vi "GetRectUnion.vi"(8 "No Error":errorcluster, 10 "B":T1, 11 "A":T1) -> (0 "Error Out":errorcluster, 3 "Union":T1)   [LabVIEW 2024, in "SDL3.lvlib" / "Rect.lvlib"]
doc: "<B>Summary</B>\nCalculate the union of two rectangles."
uses:
  Rect.lvlib
  Rect--cluster.ctl
  Lib/SDL3.dll
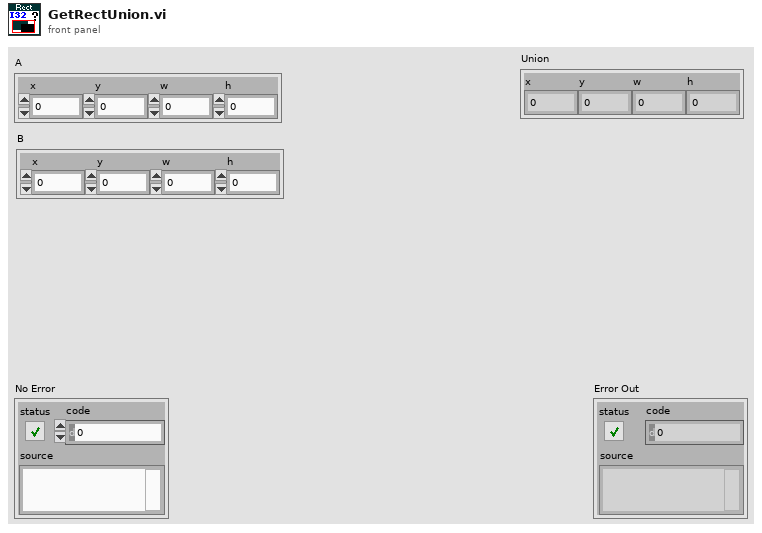
[diagram p1: front panel]
types:
  T1 = typedef "SDL3.lvlib/Rect.lvlib/Rect--cluster.ctl" = cluster{"x":i32, "y":i32, "w":i32, "h":i32}
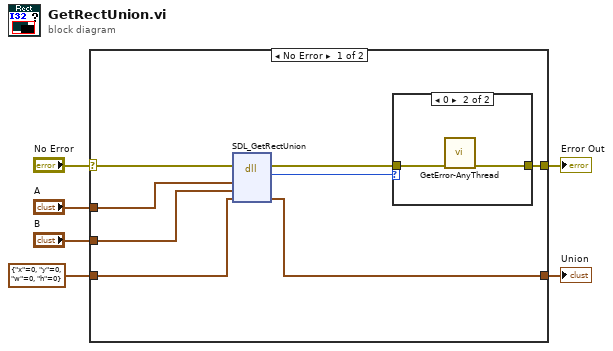
[diagram p0: block diagram]
diagram:
  n1 = case shown="No Error" "No Error" {
    selector: "No Error" -> [w14 w19]
    tunnel: "A" -> [w12 _]
    tunnel: "B" -> [w11 _]
    tunnel: [w10 w18] -> w3
    tunnel: [w9 w19] -> w2
    tunnel: T1 {"x"=0, "y"=0, "w"=0, "h"=0} ("B") -> [w7 w18]
    frame No Error {
      n2 = dll-call lib="C:/Users/Thomas/Documents/Projects/LV-SDL3/Sources/SDL3/Lib/SDL3.*" fn="SDL_GetRectUnion"(error in=w14, "A"=w12, "B"=w11, "result"=w7) -> (error out=w13:errorcluster, "return type"=w8:i32, "result"=w10:T1)  [unwired: 4 in, 1 out]
      n3 = case shown="0" w8 {
        tunnel: w13 -> [w15 w17]
        tunnel: [w15 w16] -> w9
        frame Default {
        }
        frame 0 {
          n4 = call "GetError-AnyThread.vi"("No Error"=w17) -> ("Error Out"=w16:errorcluster)  [unwired: 10 in]
        }
      }
    }
    frame Error {
    }
  }
  "Error Out" <- w2
  "Union" <- w3
